vi "Principal.vi"() -> ()   [LabVIEW 2018]
uses:
  <vilib>/vision/Instrument.llb/QR Code Stream Mode Type.ctl
  <vilib>/vision/Instrument.llb/QR Code Report.ctl
  <vilib>/vision/Instrument.llb/QR Code Model Type.ctl
  <vilib>/vision/Instrument.llb/Data Matrix Polarity.ctl
  <vilib>/vision/Instrument.llb/Demodulation Mode.ctl
  <vilib>/vision/Instrument.llb/Cell Sample Size.ctl
  <vilib>/vision/Instrument.llb/Cell Filter Mode.ctl
panel:
  out "Encontrado":bool
  out "Lectura":string
  out "Objeto compatible":bool
  out "Moviendo brazo":bool
  out "Banda activa":bool
  out "Waveform Chart":dbl(graph)
  out "error out":errorcluster
  out "QR Code Report":T1={"Found?"=FALSE, "Data"="", "Bounding Box"=[], "Errors Corrected"=0, "Dimensions (Rows/Cols)"=0, "Version"=0, "QR Model"=0, "Stream Mode"=0, "Barcode Polarity"=-2, "Mirrored?"=FALSE, "Append Stream Position"=0, "Size of Append Stream"=0, "First EAN-128 ID"=0, "First Alternate Language ID"=0, "Append Stream ID"=0, "Minimum Edge Strength"=30, "Demodulation Mode"=-2, "Cell Sample Size"=-2, "Cell Filter Mode"=-2} {"Append Stream ID" format="%x"; "Cell Filter Mode" items=["Auto-detect"=-2, "Average"=0, "Median"=1, "Central Average"=2, "High Average"=3, "Low Average"=4, "Very High Average"=5, "Very Low Average"=6, "All Filters"=8]; "Cell Sample Size" items=["Auto-detect"=-2, "1x1"=1, "2x2"=2, "3x3"=3, "4x4"=4, "5x5"=5, "6x6"=6, "7x7"=7]; "Demodulation Mode" items=["Auto-detect"=-2, "Histogram"=0, "Local Contrast"=1, "Combination"=2, "All"=3]; "Barcode Polarity" items=["Auto-detect"=-2, "Black on White"=0, "White on Black"=1]; "Stream Mode" items=["Numeric", "AlphaNumeric", "Raw Bytes", "UCC/EAN-128 - In Tokens", "UCC/EAN-128 - In Data", "Extended Character Interpretation", "Kanji"]; "QR Model" items=["Auto-detect", "Micro", "Model 1", "Model 2"]; "Version" max=40 step=1}
  out "Tokenized Output Data":T8(array[cluster]) {"Stream Mode" items=["Numeric", "AlphaNumeric", "Raw Bytes", "UCC/EAN-128 - In Tokens", "UCC/EAN-128 - In Data", "Extended Character Interpretation", "Kanji"]}
  out "Visualización":T9(plugin-control)
  in  "Parar":bool
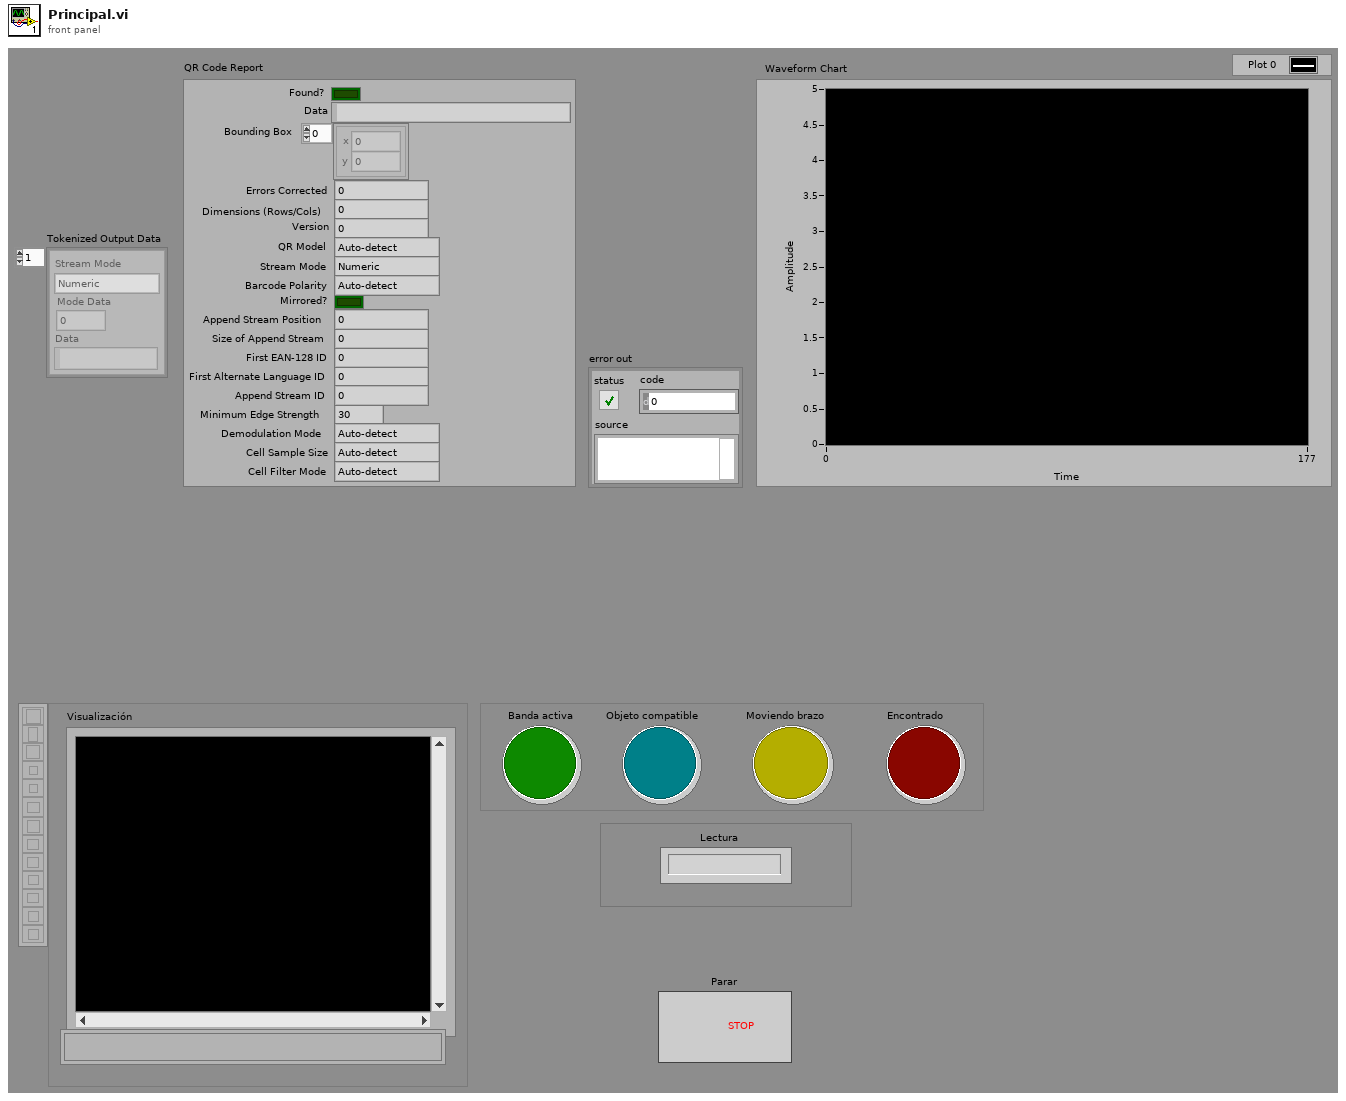
[diagram p1: front panel]
types:
  T1 = typedef "QR Code Report.ctl" = cluster{"Found?":bool, "Data":string, "Bounding Box":cluster{"x":sgl, "y":sgl}[], "Errors Corrected":u32, "Dimensions (Rows/Cols)":u32, "Version":u32, "QR Model":T2, "Stream Mode":T3, "Barcode Polarity":T4, "Mirrored?":bool, "Append Stream Position":u32, "Size of Append Stream":u32, "First EAN-128 ID":i32, "First Alternate Language ID":i32, "Append Stream ID":u32, "Minimum Edge Strength":u32, "Demodulation Mode":T5, "Cell Sample Size":T6, "Cell Filter Mode":T7}
  T2 = typedef "QR Code Model Type.ctl" = i32
  T3 = typedef "QR Code Stream Mode Type.ctl" = i32
  T4 = typedef "Data Matrix Polarity.ctl" = i32
  T5 = typedef "Demodulation Mode.ctl" = i32
  T6 = typedef "Cell Sample Size.ctl" = i32
  T7 = typedef "Cell Filter Mode.ctl" = i32
  T8 = cluster{"Stream Mode":T3, "Mode Data":u32, "Data":string}[]
  T9 = typedef "IMAQ Image.ctl" = refnum<image>
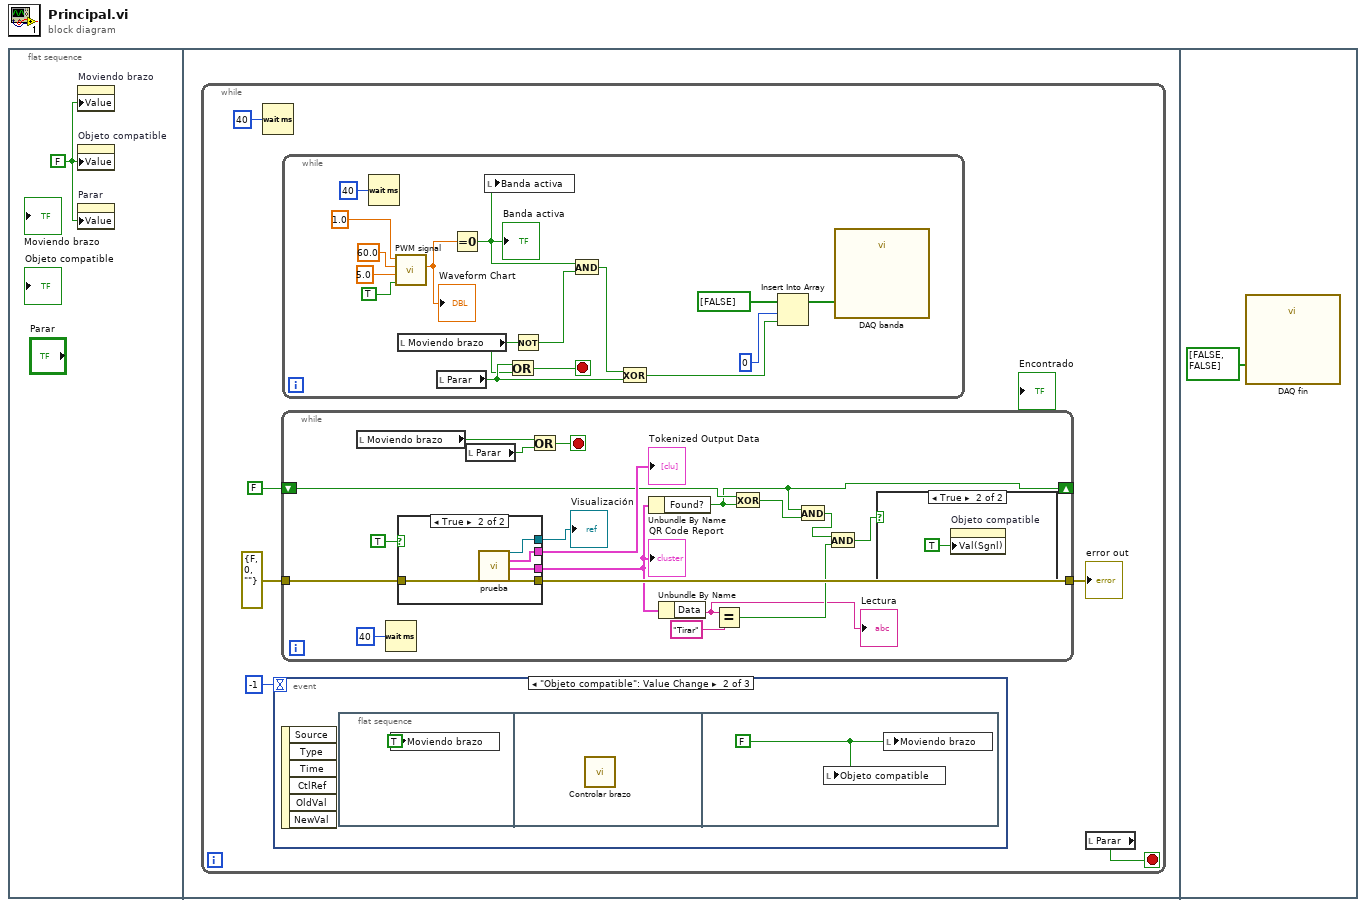
[diagram p0: block diagram]
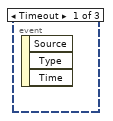
[diagram p2: hidden frame]
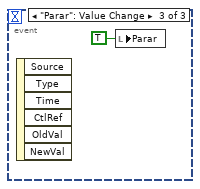
[diagram p3: hidden frame]
diagram:
  n1 = flat-sequence {
    frame #0 {
      w1 = FALSE
      n2 = property on="Moviendo brazo" class="Bool (strict)"("Value"=w1) -> ()  [unwired: 2 in, 2 out]
      n3 = property on="Objeto compatible" class="Bool (strict)"("Value"=w1) -> ()  [unwired: 2 in, 2 out]
      n4 = property on="Parar" class="Bool (strict)"("Value"=w1) -> ()  [unwired: 2 in, 2 out]
    }
    frame #1 {
      n5 = while {
        stop <- w3 stop-if-true
        n6 = Wait (ms)(milliseconds to wait=u32 40) -> ()  [unwired: 1 out]
        n7 = event shown="[1] \"Objeto compatible\": Value Change" {
          selector: _ -> [_ _ _]
          dyn-events: _ -> [_ _ _]
          timeout: -1 -> [_ _ _]
          event Timeout {
            n8 = event-data() -> ()  [unwired: 1 in, 3 out]
          }
          event "Objeto compatible": Value Change {
            n9 = event-data() -> ()  [unwired: 1 in, 6 out]
            n10 = flat-sequence {
              frame #0 {
                n11 = local write "Moviendo brazo"(TRUE) -> ()
              }
              frame #1 {
                n12 = call "Controlar brazo.vi"() -> ()  [unwired: 11 in, 1 out]
              }
              frame #2 {
                w9 = FALSE ("Control")
                n13 = local write "Objeto compatible"(w9) -> ()
                n14 = local write "Moviendo brazo"(w9) -> ()
              }
            }
          }
          event "Parar": Value Change {
            n15 = event-data() -> ()  [unwired: 1 in, 6 out]
            n16 = local write "Parar"(TRUE) -> ()
          }
        }
        n17 = while {
          tunnel: errorcluster {"status"=FALSE, "code"=0, "source"=""} ("error in") -> [w43]
          tunnel: [w42] -> w6
          shift-right: [w33] -> _
          shift-left: FALSE -> [w35]
          stop <- w38 stop-if-true
          n18 = local read "Moviendo brazo"() -> (w39:bool)
          n19 = Wait (ms)(milliseconds to wait=u32 40) -> ()  [unwired: 1 out]
          n20 = case shown="True" TRUE {
            tunnel: [_ w50] -> w44
            tunnel: [_ w49] -> w36
            tunnel: [_ w48] -> w32
            tunnel: w43 -> [_ w47]
            tunnel: [_ w46] -> w42
            frame False {
            }
            frame True {
              n21 = call "prueba.vi"("error in"=w47) -> ("Image Out"=w50:T9, "Tokenized Output Data"=w49:T8, "QR Code Report"=w48:T1, "error out"=w46:errorcluster)  [unwired: 23 in]
            }
          }
          "Visualización" <- w44
          "Tokenized Output Data" <- w36
          "QR Code Report" <- w32
          n22 = local read "Parar"() -> (w37:bool)
          n23 = Or(x=w39, y=w37) -> (x .or. y?=w38:bool)
          n24 = Unbundle By Name(w32) -> ("Found?"=w33:bool)
          n25 = Unbundle By Name(w32) -> ("Data"=w27:string)
          "Lectura" <- w27
          n26 = Equal?(x=w27, y="Tirar") -> (x = y?=w28:bool)
          n27 = Exclusive Or(1:w33, 2:w35) -> (0:w34:bool)
          n28 = And(x=w33, y=w34) -> (x .and. y?=w30:bool)
          n29 = And(x=w30, y=w28) -> (x .and. y?=w29:bool)
          n30 = case shown="True" w29 {
            frame False {
            }
            frame True {
              n31 = property on="Objeto compatible" class="Bool (strict)"("Val(Sgnl)"=TRUE ("Value (Signaling)")) -> ()  [unwired: 2 in, 2 out]
            }
          }
        }
        "error out" <- w6
        n32 = while {
          stop <- w20 stop-if-true
          n33 = Wait (ms)(milliseconds to wait=u32 40) -> ()  [unwired: 1 out]
          n34 = call "PWM signal.vi"("Signo"=TRUE, "Amplitud"=5.0, "Ciclo de trabajo"=60.0, "Frecuencia"=1.0) -> ("Waveform Chart"=w23:dbl)  [unwired: 7 in]
          "Waveform Chart" <- w23
          n35 = local read "Moviendo brazo"() -> (w14:bool)
          n36 = local read "Parar"() -> (w16:bool)
          n37 = Equal To 0?(x=w23) -> (x = 0?=w12:bool)
          "Banda activa" <- w12
          n38 = local write "Banda activa"(w12) -> ()
          n39 = Or(x=w16, y=w14) -> (x .or. y?=w20:bool)
          n40 = Not(x=w14) -> (.not. x?=w13:bool)
          n41 = And(x=w12, y=w13) -> (x .and. y?=w11:bool)
          n42 = Exclusive Or(1:w16, 2:w11) -> (0:w15:bool)
          n43 = Insert Into Array(array=bool[] [FALSE], index=0, new element=w15) -> (w17:bool[])
          n44 = call "DAQ banda"("data"=w17) -> ()  [unwired: 17 in, 2 out]
        }
        n45 = local read "Parar"() -> (w3:bool)
      }
    }
    frame #2 {
      n46 = call "DAQ fin"("data"=bool[] [FALSE, FALSE] ("array")) -> ()  [unwired: 17 in, 2 out]
    }
  }
